vi "FTW-Time-RetryTimer.vi"(0 "Retry Attempt (zero-indexed)":i32, 5 "Incremental Time to Wait (500msec)":u32=500 format="%dmsec", 11 "error in":errorcluster) -> (4 "Retry Attempt":string, 6 "Time Waited":u32 format="%dmsec", 15 "error out":errorcluster)   [LabVIEW 2013]
panel:
  # "Inputs"
  # "Outputs"
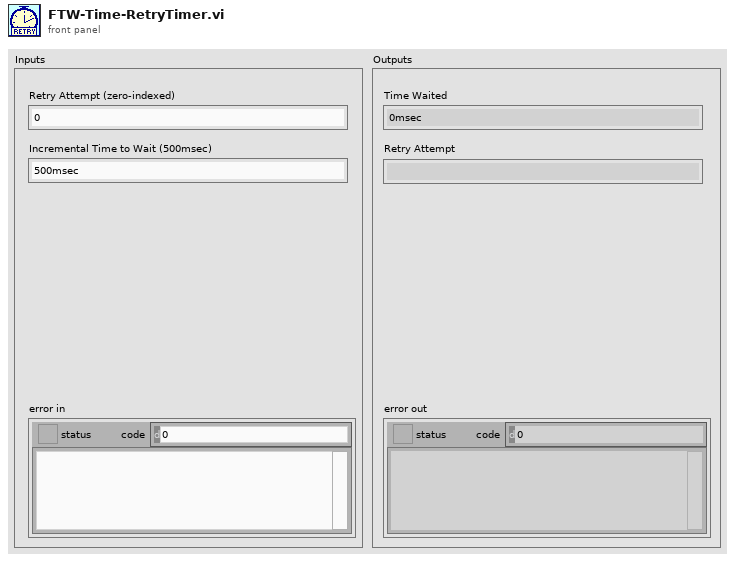
[diagram p1: front panel]
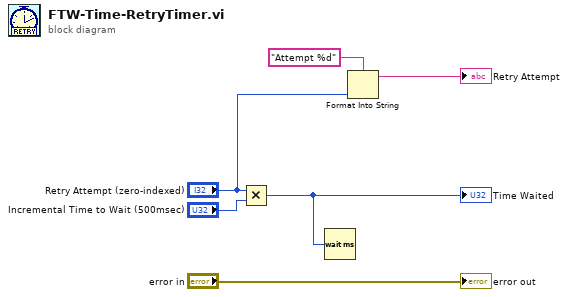
[diagram p0: block diagram]
diagram:
  n1 = Multiply(x="Retry Attempt (zero-indexed)", y="Incremental Time to Wait (500msec)") -> (x*y=w2:u32)
  "Time Waited" <- w2
  n2 = Wait (ms)(milliseconds to wait=w2) -> ()  [unwired: 1 out]
  n3 = Format Into String(format string="Attempt %d", "Retry Attempt (zero-indexed)") -> (resulting string=→"Retry Attempt":string)  [unwired: 2 in, 1 out]
  "error out" <- "error in"
